vi "CMN_inspectErros.vi"(5 "database name":string="DBS", 6 "show Dialog?":bool, 7 "message":string, 8 "error in (no error)":errorcluster, 11 "error code":i32) -> (0 "error out":errorcluster)   [LabVIEW 2016]
doc: "This subVI tests the error status output of one or more low-level functions or subVIs that output a numeric error code, and creates an error out cluster that can be wired to the Simple or General Error Handler in order to identify the error and describe it to the user.\n\nThe error in cluster is tested first. If error? is no-error, the elements of the error codes array are tested next for non-zero values. The first error found terminates the test, and error out identifies that error. Use a Build Array function to assemble the individual error codes.\n\nYou can optionally use the source messages string to pass on the source of the error. Enter one line of text for each element of the error codes array. \n\nThe error? status is TRUE on any error."
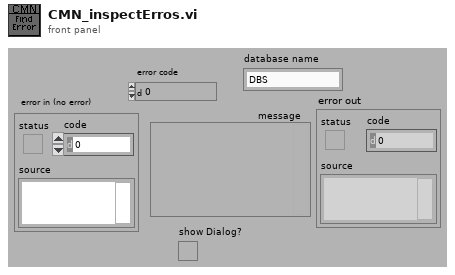
[diagram p1: front panel]
types:
  T1 = typedef "DatabaseHand_RefNum.ctl" = refnum<vi>
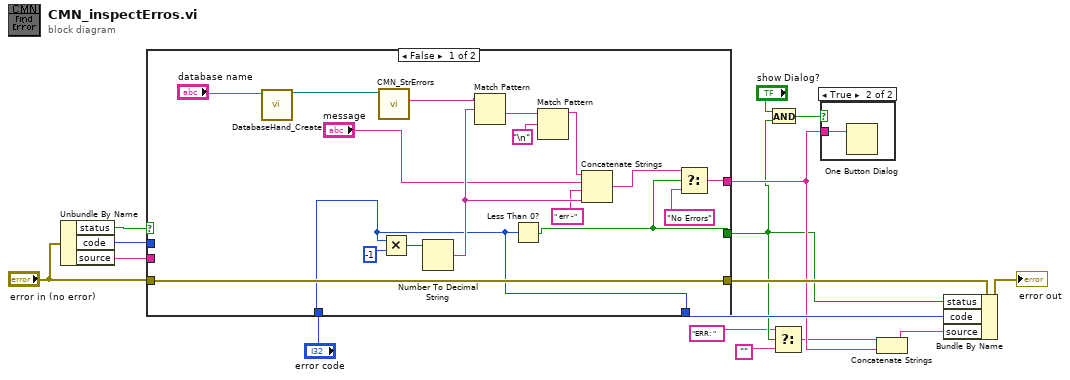
[diagram p0: block diagram]
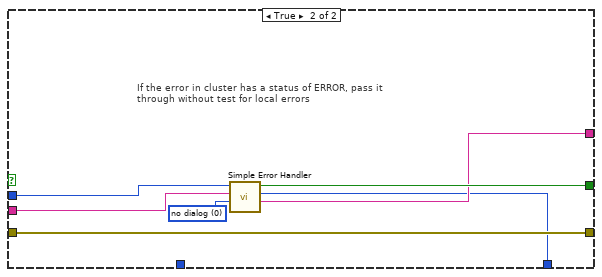
[diagram p3: hidden frame]
diagram:
  n1 = Unbundle By Name("error in (no error)") -> ("status"=w12:bool, "code"=w13:i32, "source"=w11:string)
  n2 = case shown="False" w12 {
    tunnel: "error in (no error)" -> [w33 w40]
    tunnel: [w33 w40] -> w10
    tunnel: [w22 w37] -> w6
    tunnel: [w20 w38] -> w4
    tunnel: w13 -> [_ w36]
    tunnel: w11 -> [_ w39]
    tunnel: "error code" -> [w21 _]
    tunnel: [w21 w35] -> w7
    frame False {
      n3 = call "DatabaseHand_Create.vi"("Name"="database name") -> ("Database RefNum out"=w17:T1)  [unwired: 1 in, 9 out]
      n4 = call "CMN_StrErrors.vi"("Database RefNum"=w17) -> ("errors"=w18:string)  [unwired: 10 out]
      n5 = Multiply(x=w21, y=-1) -> (x*y=w26:i32)
      n6 = Number To Decimal String(number=w26) -> (decimal integer string=w29:string)  [unwired: 1 out]
      n7 = Match Pattern(string=w18, regular expression=w29) -> (after substring=w31:string)  [unwired: 4 out]
      n8 = Less Than 0?(x=w21) -> (x < 0?=w20:bool)
      n9 = Match Pattern(string=w31, regular expression="\n") -> (before substring=w27:string)  [unwired: 4 out]
      n10 = Concatenate Strings(w27, "message", " err -", w29) -> (w23:string)
      n11 = Select(t=w23, s=w20, f="No Errors") -> (s? t:f=w22:string)
    }
    frame True {
      w34 = u16 0 items=["no dialog", "OK message", "continue or stop message"] ("type of dialog (OK msg:1)")
      # "If the error in cluster has a status of ERROR, pass it through without test for local errors"
      n12 = call <vilib>:"Simple Error Handler.vi"("error code (no error:0)"=w36, "error source (\" \")"=w39, "type of dialog (OK msg:1)"=w34) -> ("error?"=w38:bool, "code out"=w35:i32, "source out"=w37:string)  [unwired: 1 in, 3 out]
    }
  }
  n13 = And(x="show Dialog?", y=w4) -> (x .and. y?=w14:bool)
  n14 = Select(t="ERR: ", s=w4, f="") -> (s? t:f=w1:string)
  n15 = case shown="True" w14 {
    tunnel: w6 -> [_ w41]
    frame False {
    }
    frame True {
      n16 = One Button Dialog(message=w41) -> ()  [unwired: 2 out]
    }
  }
  n17 = Concatenate Strings(w1, w6) -> (w5:string)
  n18 = Bundle By Name(cluster=w10, "status"=w4, "code"=w7, "source"=w5) -> (→"error out":errorcluster)
